vi "FP Frontmost.vi"(8 "error in (no error)":errorcluster, 10 "FP Frontmost":bool=TRUE, 11 "Station Actor in":refnum<class "Station Actor.lvclass">) -> (0 "error out":errorcluster, 3 "Station Actor out":refnum<class "Station Actor.lvclass">)   [LabVIEW 2019, in "Station Actor.lvlib" / "Station Actor.lvclass"]
uses:
  Station Actor.lvclass
  Station Actor.lvclass/Station Actor.ctl
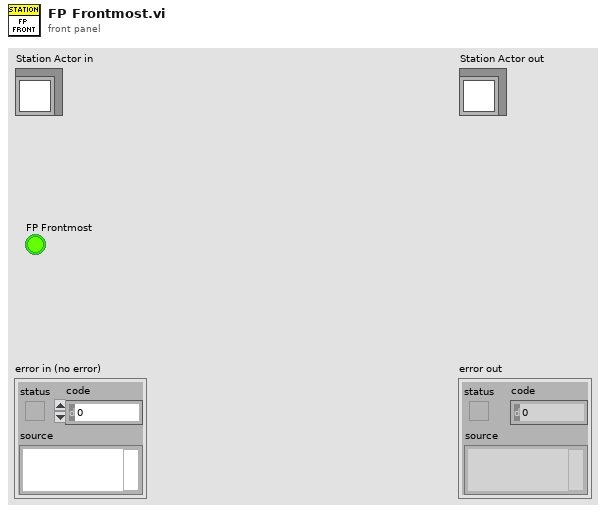
[diagram p1: front panel]
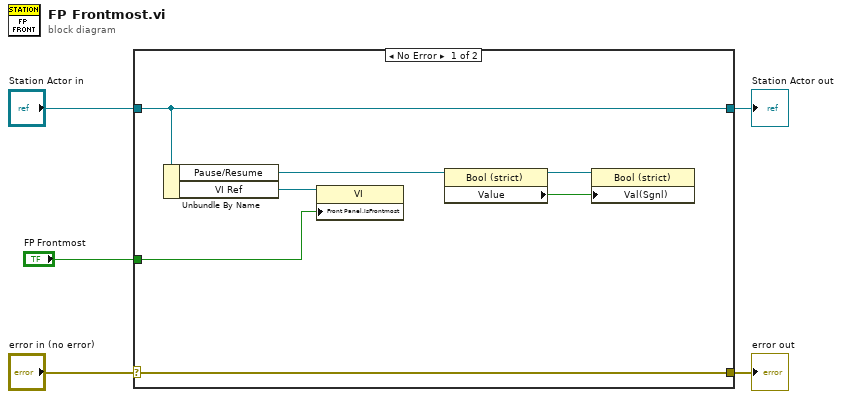
[diagram p0: block diagram]
diagram:
  n1 = case shown="No Error" "error in (no error)" {
    selector: "error in (no error)" -> [w12 w14]
    tunnel: [w12 w14] -> w4
    tunnel: [w7 w13] -> w2
    tunnel: "Station Actor in" -> [w7 w13]
    tunnel: "FP Frontmost" -> [w6 _]
    frame No Error {
      n2 = Unbundle By Name(w7) -> ("Pause/Resume"=w10:refnum<vi>, "VI Ref"=w11:refnum<vi>)
      n3 = property class="VI"(reference=w11, "Front Panel.IsFrontmost"=w6) -> ()  [unwired: 1 in, 2 out]
      n4 = property class="Bool (strict)"(reference=w10) -> (reference out=w9:refnum<vi>, "Value"=w8:bool)  [unwired: 1 in, 1 out]
      n5 = property class="Bool (strict)"(reference=w9, "Val(Sgnl)"=w8) -> ()  [unwired: 1 in, 2 out]
    }
    frame Error {
    }
  }
  "error out" <- w4
  "Station Actor out" <- w2
